vi "CalcOvrUndr.vi"(6 "StepType":string, 11 "Step Data":dbl[][][](array[numeric])) -> (1 "StepData":dbl[][][](array[numeric]), 2 "StepSize":dbl[][](array[numeric]), 3 "OvrUndr":dbl[][][](array[numeric]))   [LabVIEW 2014]
uses:
  <vilib>/Analysis/NI_AALBase.lvlib
panel:
  # "IA"
  # "VA"
  # "VB"
  # "VC"
  # "V+"
  # "IB"
  # "IC"
  # "I+"
  # "PreOvr"
  # "PreUndr"
  # "PostOvr"
  # "PostUndr"
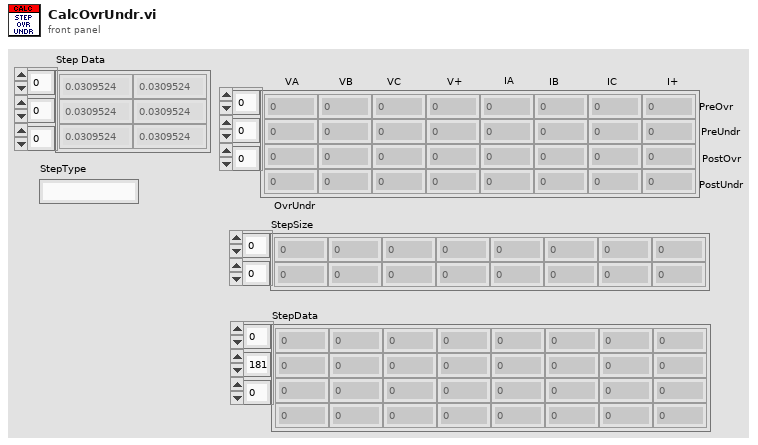
[diagram p1: front panel]
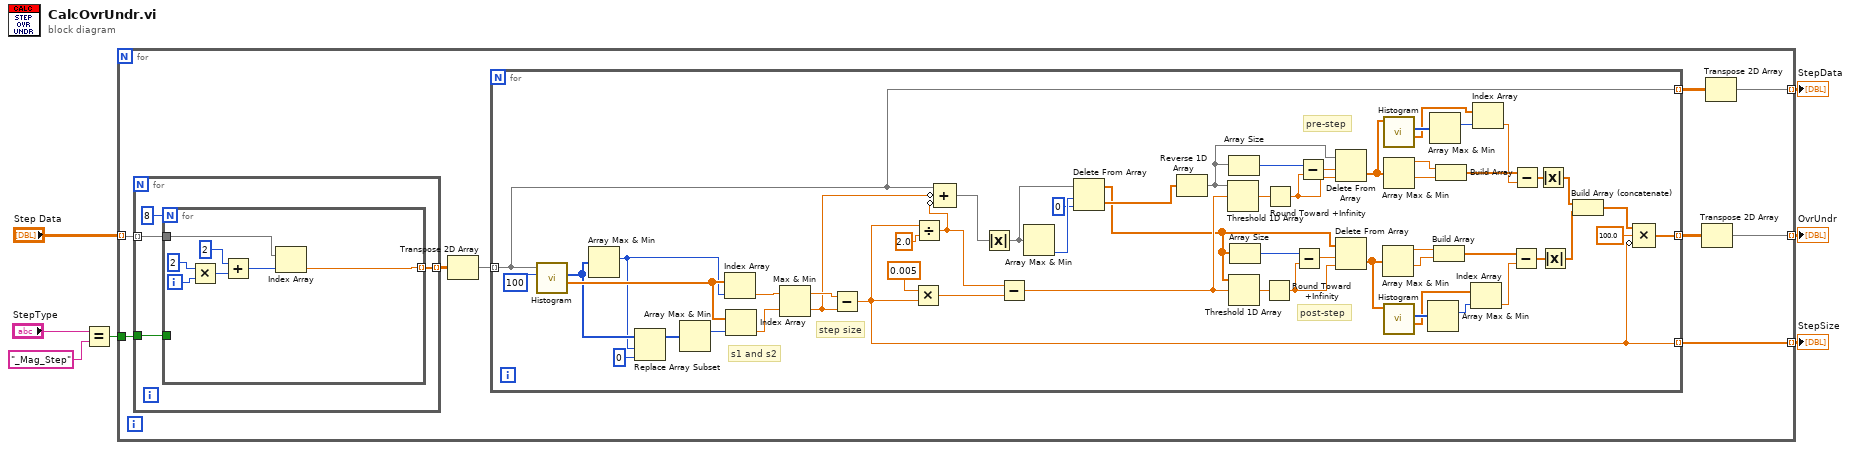
[diagram p0: block diagram]
diagram:
  n1 = Equal?(x="StepType", y="_Mag_Step") -> (x = y?=w4:bool)
  n2 = for {
    tunnel: "Step Data" -> [w16] mode=indexing
    tunnel: w4 -> [w15]
    tunnel: [w11] -> w3 mode=indexing
    tunnel: [w10] -> w2 mode=indexing
    tunnel: [w9] -> w1 mode=indexing
    n3 = for {
      tunnel: w16 -> [w76] mode=indexing
      tunnel: [w75] -> w14 mode=indexing
      tunnel: w15 -> [w74]
      n4 = for {
        N: 8 -> [_]
        tunnel: w76 -> [w78]
        tunnel: [w77] -> w75 mode=indexing
        tunnel: w74 -> [_]
        i -> [w83]
        n5 = Multiply(x=2, y=w83) -> (x*y=w81:i32)
        n6 = Add(x=2, y=w81) -> (x+y=w79:i32)
        n7 = Index Array(array=w78, index=w79) -> (element=w77:dbl)
      }
    }
    n8 = Transpose 2D Array(2D array=w14) -> (transposed array=w13:dbl[][])
    n9 = for {
      tunnel: w13 -> [w25] mode=indexing
      tunnel: [w28] -> w12 mode=indexing
      tunnel: [w26] -> w10 mode=indexing
      tunnel: [w25] -> w8 mode=indexing
      # "post-step"
      # "pre-step"
      # "step size"
      # "s1 and s2"
      n10 = call <vilib>:"Histogram.vi"("intervals"=100, "X"=w25) -> ("X Values"=w71:dbl[], "Histogram: h(x)"=w57:i32[])  [unwired: 6 in, 2 out]
      n11 = Array Max & Min(array=w57) -> (max index (indices)=w56:i32)  [unwired: 3 out]
      n12 = Replace Array Subset(array=w57, new element=0 ("new element/subarray"), index=w56) -> (w54:i32[])
      n13 = Array Max & Min(array=w54) -> (max index (indices)=w53:i32)  [unwired: 3 out]
      n14 = Index Array(array=w71, index=w56) -> (element=w52:dbl)
      n15 = Index Array(array=w71, index=w53) -> (element=w51:dbl)
      n16 = Max & Min(x=w52, y=w51) -> (max(x,y)=w50:dbl, min(x,y)=w49:dbl)
      n17 = Subtract(x=w50, y=w49) -> (x-y=w26:dbl)
      n18 = Multiply(x=0.005, y=w26) -> (x*y=w69:dbl)
      n19 = Divide(x=w26, y=2.0) -> (x/y=w48:dbl)
      n20 = Compound Arithmetic op=ADD(w25, invert w49, invert w48) -> (w21:dbl[])
      n21 = Absolute Value(x=w21) -> (abs(x)=w22:dbl[])
      n22 = Subtract(x=w48, y=w69) -> (x-y=w68:dbl)
      n23 = Array Max & Min(array=w22) -> (min index (indices)=w20:i32)  [unwired: 3 out]
      n24 = Delete From Array(array=w22, length=w20, index=0) -> (deleted portion=w18:dbl[], array with subset deleted=w17:dbl[])
      n25 = Reverse 1D Array(array=w18) -> (reversed array=w59:dbl[])
      n26 = Threshold 1D Array(2:w68, 3:w59) -> (0:w67:dbl)  [unwired: 1 in]
      n27 = Array Size(array=w59) -> (size(s)=w62:i32)
      n28 = Threshold 1D Array(2:w68, 3:w17) -> (0:w66:dbl)  [unwired: 1 in]
      n29 = Array Size(array=w17) -> (size(s)=w65:i32)
      n30 = Round Toward +Infinity(x=w66) -> (ceil(x): smallest int >= x=w63:dbl)
      n31 = Round Toward +Infinity(x=w67) -> (ceil(x): smallest int >= x=w60:dbl)
      n32 = Subtract(x=w65, y=w63) -> (x-y=w64:dbl)
      n33 = Subtract(x=w62, y=w60) -> (x-y=w61:dbl)
      n34 = Delete From Array(array=w59, length=w61, index=w60) -> (deleted portion=w24:dbl[])  [unwired: 1 out]
      n35 = Delete From Array(array=w17, length=w64, index=w63) -> (deleted portion=w23:dbl[])  [unwired: 1 out]
      n36 = Array Max & Min(array=w23) -> (max value=w39:dbl, min value=w38:dbl)  [unwired: 2 out]
      n37 = call <vilib>:"Histogram.vi"("X"=w24) -> ("X Values"=w44:dbl[], "Histogram: h(x)"=w47:i32[])  [unwired: 7 in, 2 out]
      n38 = Array Max & Min(array=w24) -> (max value=w41:dbl, min value=w42:dbl)  [unwired: 2 out]
      n39 = call <vilib>:"Histogram.vi"("X"=w23) -> ("X Values"=w43:dbl[], "Histogram: h(x)"=w46:i32[])  [unwired: 7 in, 2 out]
      n40 = Array Max & Min(array=w46) -> (max index (indices)=w27:i32)  [unwired: 3 out]
      n41 = Array Max & Min(array=w47) -> (max index (indices)=w45:i32)  [unwired: 3 out]
      n42 = Build Array(w39, w38) -> (w37:dbl[])
      n43 = Build Array(w41, w42) -> (w34:dbl[])
      n44 = Index Array(array=w43, index=w27) -> (element=w36:dbl)
      n45 = Index Array(array=w44, index=w45) -> (element=w33:dbl)
      n46 = Subtract(x=w37, y=w36) -> (x-y=w35:dbl[])
      n47 = Subtract(x=w34, y=w33) -> (x-y=w32:dbl[])
      n48 = Absolute Value(x=w32) -> (abs(x)=w31:dbl[])
      n49 = Absolute Value(x=w35) -> (abs(x)=w30:dbl[])
      n50 = Build Array (concatenate)(w31, w30) -> (w29:dbl[])
      n51 = Compound Arithmetic op=MULTIPLY(w29, 100.0, invert w26) -> (w28:dbl[])
    }
    n52 = Transpose 2D Array(2D array=w12) -> (transposed array=w11:dbl[][])
    n53 = Transpose 2D Array(2D array=w8) -> (transposed array=w9:dbl[][])
  }
  "OvrUndr" <- w3
  "StepSize" <- w2
  "StepData" <- w1
